vi "Read Digital Inputs.vi"(8 "error in (no error)":errorcluster, 9 "Device Number":string, 11 "VISA resource name":refnum<visa-resource-name>) -> (0 "error out":errorcluster, 1 "Digital Input Pins":bool[](array[boolean]), 3 "VISA resource name out":refnum<visa-resource-name>)   [LabVIEW 2015, in "Zaber A Series.lvlib"]
doc: "Reads the digital input pins on Zaber devices that have them. Produces an array of booleans containing one entry for each input pin.\n \nThis VI requires that the Initialize VI has been called with the same serial port."
uses:
  Zaber A Series.lvlib
  Private/All Commands.ctl
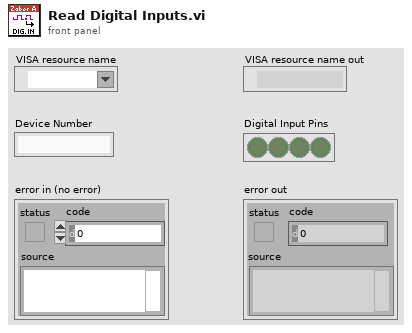
[diagram p1: front panel]
types:
  T1 = typedef "Zaber A Series.lvlib/All Commands.ctl" = string
  T2 = cluster{"Device":string, "Axis":string, "Reply Flag":string, "Status":string, "Warning Flags":string, "Data":string}
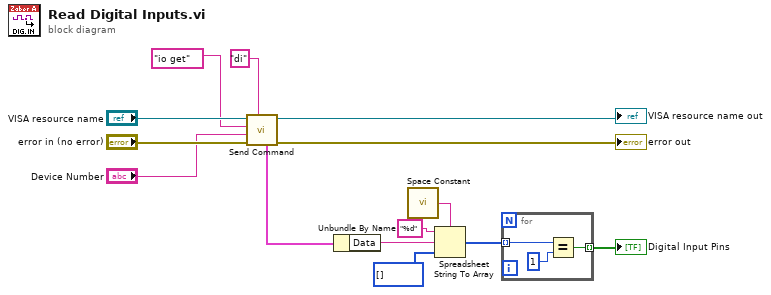
[diagram p0: block diagram]
diagram:
  n1 = call "Send Command.vi"("Data"="di", "error in (no error)"="error in (no error)", "Device and Axis"="Device Number", "Command"=T1 "io get" ("Complete Command List"), "VISA resource name"="VISA resource name") -> ("error out"=→"error out":errorcluster, "VISA resource name out"=→"VISA resource name out":refnum<visa-resource-name>, "First Response Bundle"=w1:T2)  [unwired: 1 in, 3 out]
  n2 = Unbundle By Name(w1) -> ("Data"=w8:string)
  n3 = call <vilib>:"Space Constant.vi"() -> ("String"=w10:string)
  n4 = Spreadsheet String To Array(delimiter (Tab)=w10, format string="%d", spreadsheet string=w8, array type (2D Dbl)=i32[] []) -> (array=w6:i32[])
  n5 = for {
    tunnel: [w17] -> w5 mode=indexing
    tunnel: w6 -> [w16] mode=indexing
    n6 = Equal?(x=w16, y=1 ("x")) -> (x = y?=w17:bool)
  }
  "Digital Input Pins" <- w5
